vi "Calibrate.vi"(8 "error in (no error)":errorcluster, 10 "Energy":dbl[unit], 11 "HIJ Vision App Fluence and Energy Camera in":refnum<class "HIJ Vision App Fluence and Energy Camera.lvclass">) -> (0 "error out":errorcluster, 3 "HIJ Vision App Fluence and Energy Camera out":refnum<class "HIJ Vision App Fluence and Energy Camera.lvclass">)   [LabVIEW 2014, in "HIJ Vision App Fluence and Energy Camera.lvlib" / "HIJ Vision App Fluence and Energy Camera.lvclass"]
uses:
  HIJ Vision App Fluence and Energy Camera.lvclass
  Analyze/Analyze Parameter/Analyze Parameter Energy per Count/Analyze Parameter Energy per Count.lvclass
  HIJ Vision App Fluence and Energy Camera.lvclass/HIJ Vision App Fluence and Energy Camera.ctl
  Analyze/Analyze Parameter/Analyze Parameter Energy per Count/Analyze Parameter Energy per Count.lvclass/Analyze Parameter Energy per Count.ctl
  Analyze/Analyze Parameter/Analyze Parameter Energy per Count/Write J_count.vi
  HIJ Vision Application/HIJ Vision Application/HIJ Vision Application.lvclass
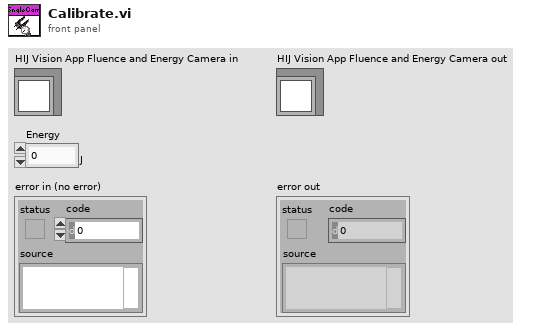
[diagram p1: front panel]
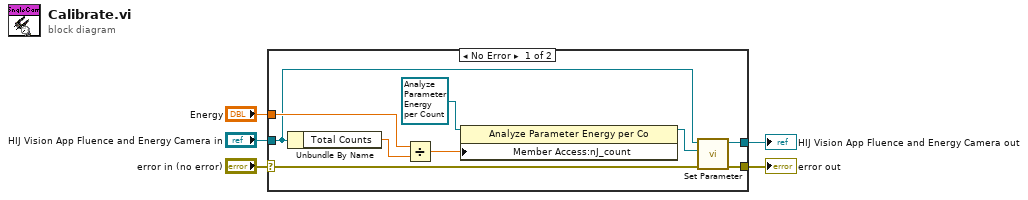
[diagram p0: block diagram]
diagram:
  n1 = case shown="No Error" "error in (no error)" {
    selector: "error in (no error)" -> [w7 w16]
    tunnel: [w6 w16] -> w4
    tunnel: [w9 w15] -> w2
    tunnel: "HIJ Vision App Fluence and Energy Camera in" -> [w10 w15]
    tunnel: "Energy" -> [w13 _]
    frame No Error {
      n2 = Unbundle By Name(w10) -> ("Total Counts"=w14:dbl)
      n3 = Divide(x=w13, y=w14) -> (x/y=w11:dbl[unit])
      n4 = property class="Analyze Parameter Energy per Co"(reference=refnum<class "Analyze Parameter Energy per Count.lvclass"> refnum ("Analyze Parameter Energy per Count.lvclass"), "Member Access:nJ_count"=w11) -> (reference out=w8:refnum<class "Analyze Parameter Energy per Count.lvclass">)  [unwired: 1 in, 1 out]
      n5 = call "Set Parameter.vi"("error in (no error)"=w7, "Parameter"=w8, "HIJ Vision Application in"=w10) -> ("error out"=w6:errorcluster, "HIJ Vision Application out"=w9:refnum<class "HIJ Vision App Fluence and Energy Camera.lvclass">)  [unwired: 7 in]
    }
    frame Error {
    }
  }
  "error out" <- w4
  "HIJ Vision App Fluence and Energy Camera out" <- w2
